vi "parseDataMotev2.vi"(0 "input data":string) -> (1 "source type (1 byte)":u8, 2 "node id (1 byte)":u8, 3 "data 1 (2 bytes)":u16, 4 "data 2 (2 bytes)":u16, 5 "data 3 (2 bytes)":u16, 6 "data 4 (2 bytes)":u16)   [LabVIEW 2011]
panel:
  out "input data size (in bytes)":i32
  out "input data (in hex)":string[](array[string])
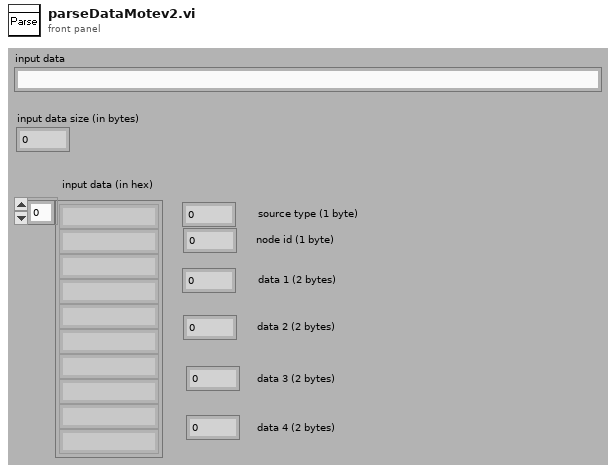
[diagram p1: front panel]
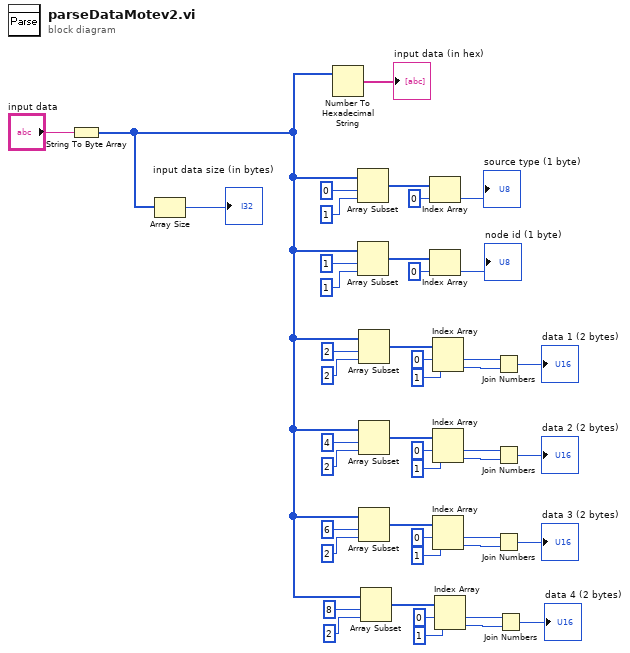
[diagram p0: block diagram]
diagram:
  n1 = String To Byte Array(string="input data") -> (unsigned byte array=w2:u8[])
  n2 = Array Size(array=w2) -> (size(s)=→"input data size (in bytes)":i32)
  n3 = Number To Hexadecimal String(2:w2) -> (0:→"input data (in hex)":string[])  [unwired: 1 in]
  n4 = Array Subset(array=w2, index=0 ("x"), length=1 ("x")) -> (w39:u8[])
  n5 = Array Subset(array=w2, index=1 ("x"), length=1 ("x")) -> (w33:u8[])
  n6 = Array Subset(array=w2, index=2 ("x"), length=2 ("x")) -> (w36:u8[])
  n7 = Array Subset(array=w2, index=4 ("x"), length=2 ("x")) -> (w25:u8[])
  n8 = Array Subset(array=w2, index=6 ("x"), length=2 ("x")) -> (w17:u8[])
  n9 = Array Subset(array=w2, index=8 ("x"), length=2 ("x")) -> (w5:u8[])
  n10 = Index Array(array=w39, index=0) -> (element=→"source type (1 byte)":u8)
  n11 = Index Array(array=w33, index=0) -> (element=→"node id (1 byte)":u8)
  n12 = Index Array(array=w36, index #1=0 ("index"), index #2=1 ("index")) -> (element #1=w30:u8, element #2=w29:u8)
  n13 = Index Array(array=w25, index #1=0 ("index"), index #2=1 ("index")) -> (element #1=w22:u8, element #2=w21:u8)
  n14 = Index Array(array=w17, index #1=0 ("index"), index #2=1 ("index")) -> (element #1=w14:u8, element #2=w13:u8)
  n15 = Index Array(array=w5, index #1=0 ("index"), index #2=1 ("index")) -> (element #1=w8:u8, element #2=w9:u8)
  n16 = Join Numbers(hi=w30, lo=w29) -> ((hi.lo)=→"data 1 (2 bytes)":u16)
  n17 = Join Numbers(hi=w22, lo=w21) -> ((hi.lo)=→"data 2 (2 bytes)":u16)
  n18 = Join Numbers(hi=w14, lo=w13) -> ((hi.lo)=→"data 3 (2 bytes)":u16)
  n19 = Join Numbers(hi=w8, lo=w9) -> ((hi.lo)=→"data 4 (2 bytes)":u16)
